vi "Find Channel.vi"(0 "SigMan in":refnum<class "SignalManager.lvclass">, 7 "regular expression":string, 11 "error in (no error)":errorcluster) -> (4 "SigMan out":refnum<class "SignalManager.lvclass">, 6 "Channel":refnum<class "Channel.lvclass">, 10 "found":bool, 15 "error out":errorcluster)   [LabVIEW 2015, in "SignalManager.lvclass"]
uses:
  SignalManager.lvclass
  Channel/Channel.lvclass
  SignalManager.lvclass/SignalManager.ctl
  Channel/Channel.lvclass/Channel.ctl
  Channel/Read Destination.vi
  <vilib>/regexp/Match Regular Expression.xnode
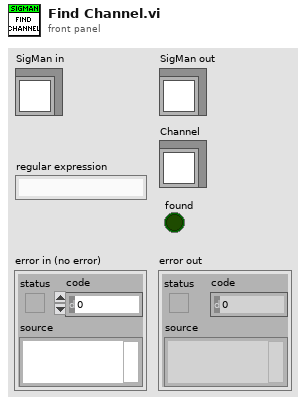
[diagram p1: front panel]
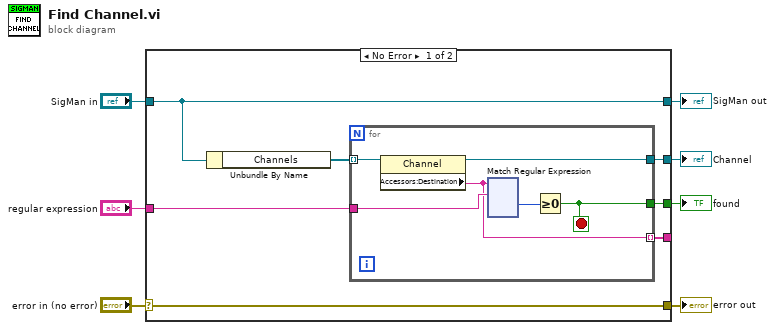
[diagram p0: block diagram]
diagram:
  n1 = case shown="No Error" "error in (no error)" {
    selector: "error in (no error)" -> [w14 w136]
    tunnel: [w14 w136] -> w6
    tunnel: [w13 w135] -> w4
    tunnel: "SigMan in" -> [w13 w135]
    tunnel: "regular expression" -> [w11 _]
    tunnel: [w10 _] -> w2
    tunnel: [w9 _] -> w1
    tunnel: [w8 _] -> _
    frame No Error {
      n2 = Unbundle By Name(w13) -> ("Channels"=w12:refnum<class "Channel.lvclass">[])
      n3 = for {
        tunnel: w12 -> [w20] mode=indexing
        tunnel: w11 -> [w19]
        tunnel: [w17] -> w9
        tunnel: [w16] -> w10
        tunnel: [w15] -> w8 mode=indexing
        stop <- w16 stop-if-true
        n4 = property class="Channel"(reference=w20) -> (reference out=w17:refnum<class "Channel.lvclass">, "Accessors:Destination"=w15:string)  [unwired: 1 in, 1 out]
        n5 = xnode "Match Regular Expression"("input string"=w15, "regular expression"=w19) -> ("offset past match"=w18:i32)  [unwired: 4 in, 4 out]
        n6 = Greater Or Equal To 0?(x=w18) -> (x >= 0?=w16:bool)
      }
    }
    frame Error {
    }
  }
  "error out" <- w6
  "SigMan out" <- w4
  "found" <- w2
  "Channel" <- w1
